vi "9_Maint_u_2.vi"() -> ()   [LabVIEW 2011]
uses:
  Globals/Global VI.vi
panel:
  in  "Process Stop Button":bool
  # "Maintenance"
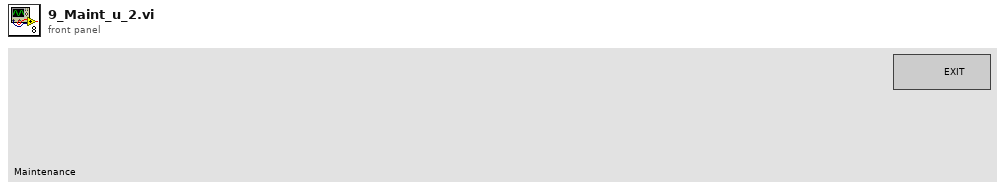
[diagram p1: front panel]
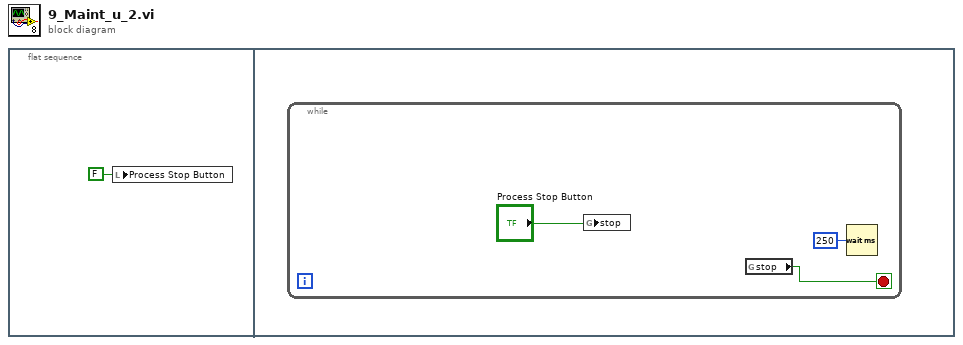
[diagram p0: block diagram]
diagram:
  n1 = flat-sequence {
    frame #0 {
      n2 = local write "Process Stop Button"(FALSE ("Process Stop Button")) -> ()
    }
    frame #1 {
      n3 = while {
        stop <- w3 stop-if-true
        n4 = global write "Global VI.vi" "stop"("Process Stop Button") -> ()
        n5 = global read "Global VI.vi" "stop"() -> (w3:bool)
        n6 = Wait (ms)(milliseconds to wait=u32 250) -> ()  [unwired: 1 out]
      }
    }
  }
